vi "to string array.vi"(8 "error in (no error)":errorcluster, 11 "module configuration in":refnum<class "Daqmx Module configuration.lvclass">) -> (0 "error out":errorcluster, 1 "Array":string[][](array[string]), 2 "version":string, 3 "module configuration out":refnum<class "Daqmx Module configuration.lvclass">)   [LabVIEW 2014, in "DAQmx Module Configuration.lvclass"]
uses:
  Daqmx Module configuration.lvclass
  Daqmx Module configuration.lvclass/Daqmx Module configuration.ctl
  <vilib>/NI/Tag Bus/tag/tag descriptor.lvclass/tag descriptor.ctl
  <vilib>/NI/Tag Bus Module Framework/module configuration/TBM module configuration.lvclass
  <vilib>/NI/Tag Bus/tag/tag descriptor.lvclass
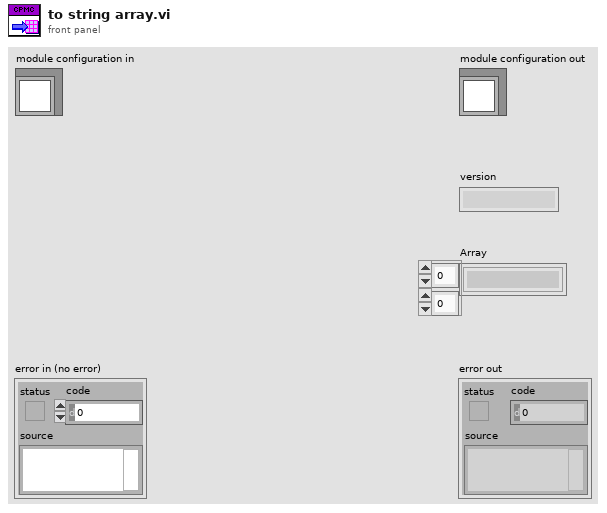
[diagram p1: front panel]
types:
  T1 = typedef "DAQmx Module Configuration.lvclass/Line.ctl" = cluster{"channel":refnum<class "TBM channel.lvclass">, "Physical Channel":string, "Measurement Type":T2, "Parameters":T3}
  T2 = typedef "DAQmx Module Configuration.lvclass/Measurement Type.ctl" = enum16{"Digital Input", "Digital Output", "Voltage Input", "Voltage Output", "Current Input", "Current Output", "RTD", "Thermocouple", "Strain"}
  T3 = typedef "DAQmx Module Configuration.lvclass/Parameters.ctl" = cluster{"Digital Config":cluster{"Invert Lines?":bool}, "Voltage Config":cluster{"Maximum Value (V)":dbl, "Minimum Value (V)":dbl, "in terminal configuration (V)":i32, "out terminal configuration (V)":i32}, "Current Config":cluster{"Maximum Value (A)":dbl, "Minimum Value (A)":dbl, "shunt resistor location":i32, "input terminal configuration (C)":i32, "external shunt resistor value":dbl}, "RTD Config":cluster{"Maximum Value (°C)":dbl, "Minimum Value (°C)":dbl, "resistance configuration":i32, "r0":dbl, "current excitation value":dbl, "rtd type":i32, "current excitation source":i32}, "Thermocouple Config":cluster{"Minimum Value (C)":dbl, "Maximum Value (C)":dbl, "thermocouple type":i32, "cjc source":i32, "cjc value":dbl}, "Strain Config":cluster{"Maximum Value":dbl, "Minimum Value":dbl, "bridge information":cluster{"strain configuration":i32, "lead wire resistance":dbl, "initial bridge voltage":dbl, "voltage excitation source":i32, "voltage excitation value":dbl}, "strain gage information":cluster{"gage factor":dbl, "nominal gage resistance":dbl, "poisson ratio":dbl}}}
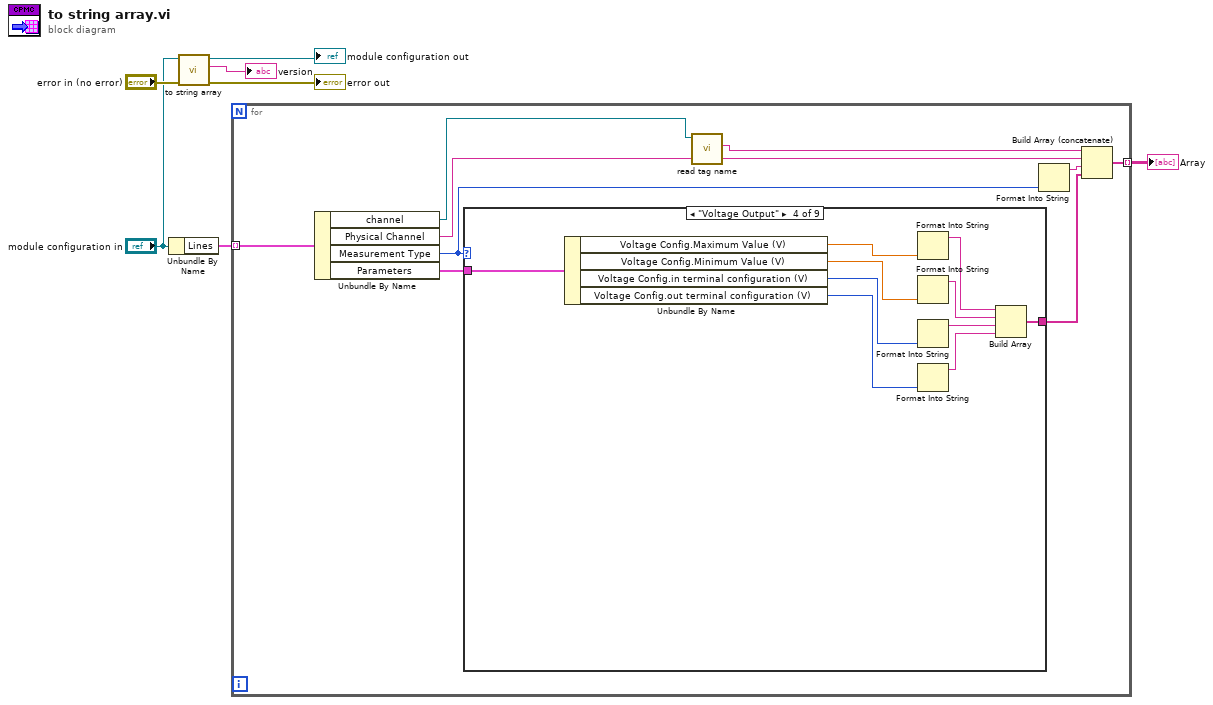
[diagram p0: block diagram]
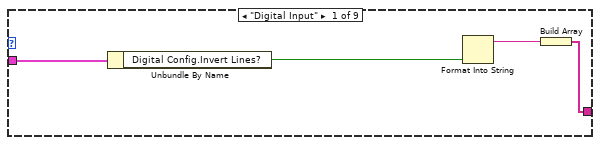
[diagram p2: hidden frame]
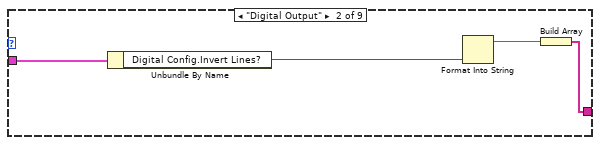
[diagram p3: hidden frame]
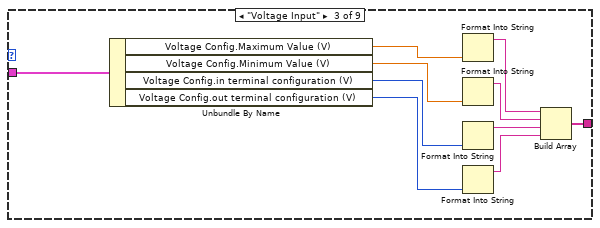
[diagram p4: hidden frame]
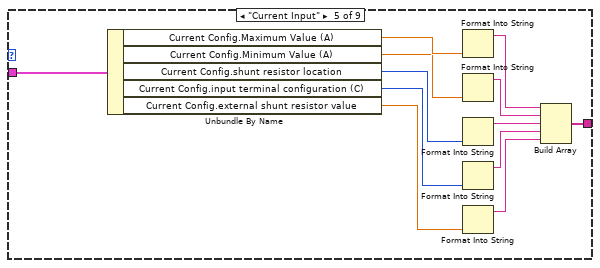
[diagram p5: hidden frame]
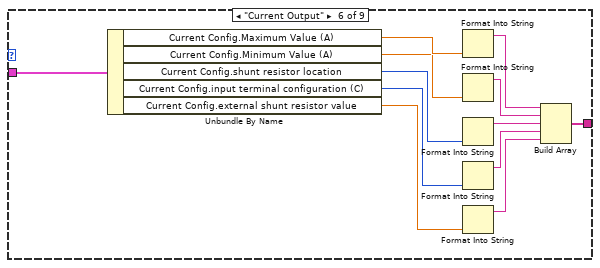
[diagram p6: hidden frame]
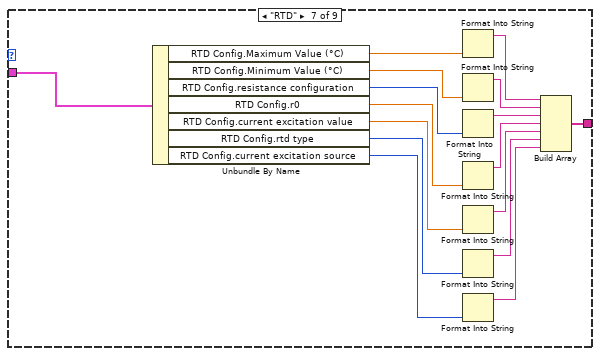
[diagram p7: hidden frame]
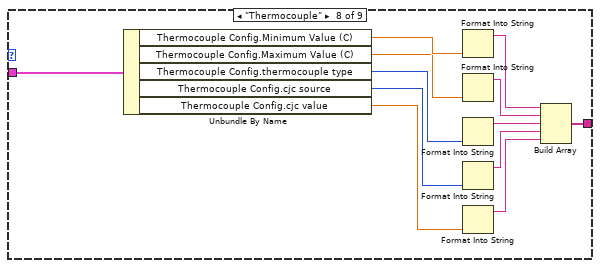
[diagram p8: hidden frame]
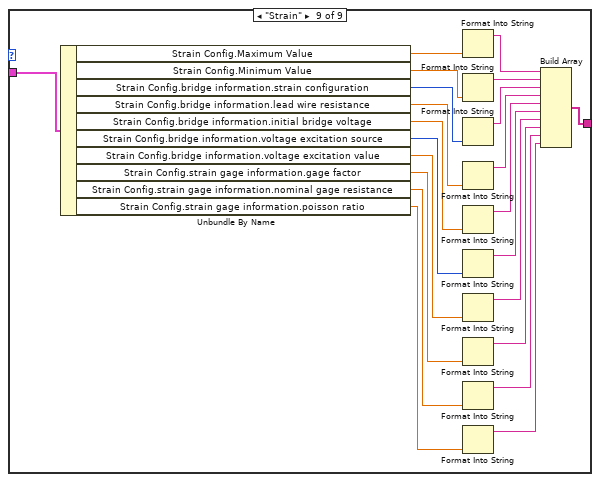
[diagram p9: hidden frame]
diagram:
  n1 = Unbundle By Name("module configuration in") -> ("Lines"=w2:T1[])
  n2 = call-parent "to string array.vi"("error in (no error)"="error in (no error)", "module configuration in"="module configuration in") -> ("error out"=→"error out":errorcluster, "version"=→"version":string, "module configuration out"=→"module configuration out":refnum<class "Daqmx Module configuration.lvclass">)  [unwired: 6 in, 1 out]
  n3 = for {
    tunnel: [w13] -> w1 mode=indexing
    tunnel: w2 -> [w16] mode=indexing
    n4 = Unbundle By Name(w16) -> ("channel"=w9:refnum<class "TBM channel.lvclass">, "Physical Channel"=w15:string, "Measurement Type"=w12:T2, "Parameters"=w11:T3)
    n5 = case shown="\"Voltage Output\"" w12 {
      tunnel: w11 -> [w20 w24 w34 w44 w56 w68 w84 w96 w118]
      tunnel: [w17 w21 w31 w41 w53 w65 w81 w93 w115] -> w10
      frame "Digital Input" {
        n6 = Unbundle By Name(w20) -> ("Digital Config.Invert Lines?"=w19:bool)
        n7 = Format Into String(w19) -> (resulting string=w18:string)  [unwired: 3 in, 1 out]
        n8 = Build Array(w18) -> (w17:string[])
      }
      frame "Digital Output" {
        n9 = Unbundle By Name(w24) -> ("Digital Config.Invert Lines?"=w23:bool)
        n10 = Format Into String(w23) -> (resulting string=w22:string)  [unwired: 3 in, 1 out]
        n11 = Build Array(w22) -> (w21:string[])
      }
      frame "Voltage Input" {
        n12 = Unbundle By Name(w34) -> ("Voltage Config.Maximum Value (V)"=w33:dbl, "Voltage Config.Minimum Value (V)"=w27:dbl, "Voltage Config.in terminal configuration (V)"=w26:i32, "Voltage Config.out terminal configuration (V)"=w25:i32)
        n13 = Format Into String(w33) -> (resulting string=w32:string)  [unwired: 3 in, 1 out]
        n14 = Format Into String(w27) -> (resulting string=w30:string)  [unwired: 3 in, 1 out]
        n15 = Format Into String(w26) -> (resulting string=w29:string)  [unwired: 3 in, 1 out]
        n16 = Format Into String(w25) -> (resulting string=w28:string)  [unwired: 3 in, 1 out]
        n17 = Build Array(w32, w30, w29, w28) -> (w31:string[])
      }
      frame "Voltage Output" {
        n18 = Unbundle By Name(w44) -> ("Voltage Config.Maximum Value (V)"=w43:dbl, "Voltage Config.Minimum Value (V)"=w37:dbl, "Voltage Config.in terminal configuration (V)"=w36:i32, "Voltage Config.out terminal configuration (V)"=w35:i32)
        n19 = Format Into String(w43) -> (resulting string=w42:string)  [unwired: 3 in, 1 out]
        n20 = Format Into String(w37) -> (resulting string=w40:string)  [unwired: 3 in, 1 out]
        n21 = Format Into String(w36) -> (resulting string=w39:string)  [unwired: 3 in, 1 out]
        n22 = Format Into String(w35) -> (resulting string=w38:string)  [unwired: 3 in, 1 out]
        n23 = Build Array(w42, w40, w39, w38) -> (w41:string[])
      }
      frame "Current Input" {
        n24 = Unbundle By Name(w56) -> ("Current Config.Maximum Value (A)"=w55:dbl, "Current Config.Minimum Value (A)"=w49:dbl, "Current Config.shunt resistor location"=w50:i32, "Current Config.input terminal configuration (C)"=w51:i32, "Current Config.external shunt resistor value"=w52:dbl)
        n25 = Format Into String(w55) -> (resulting string=w54:string)  [unwired: 3 in, 1 out]
        n26 = Format Into String(w49) -> (resulting string=w48:string)  [unwired: 3 in, 1 out]
        n27 = Format Into String(w50) -> (resulting string=w47:string)  [unwired: 3 in, 1 out]
        n28 = Format Into String(w51) -> (resulting string=w46:string)  [unwired: 3 in, 1 out]
        n29 = Format Into String(w52) -> (resulting string=w45:string)  [unwired: 3 in, 1 out]
        n30 = Build Array(w54, w48, w47, w46, w45) -> (w53:string[])
      }
      frame "Current Output" {
        n31 = Unbundle By Name(w68) -> ("Current Config.Maximum Value (A)"=w67:dbl, "Current Config.Minimum Value (A)"=w61:dbl, "Current Config.shunt resistor location"=w62:i32, "Current Config.input terminal configuration (C)"=w63:i32, "Current Config.external shunt resistor value"=w64:dbl)
        n32 = Format Into String(w67) -> (resulting string=w66:string)  [unwired: 3 in, 1 out]
        n33 = Format Into String(w61) -> (resulting string=w60:string)  [unwired: 3 in, 1 out]
        n34 = Format Into String(w62) -> (resulting string=w59:string)  [unwired: 3 in, 1 out]
        n35 = Format Into String(w63) -> (resulting string=w58:string)  [unwired: 3 in, 1 out]
        n36 = Format Into String(w64) -> (resulting string=w57:string)  [unwired: 3 in, 1 out]
        n37 = Build Array(w66, w60, w59, w58, w57) -> (w65:string[])
      }
      frame "RTD" {
        n38 = Unbundle By Name(w84) -> ("RTD Config.Maximum Value (°C)"=w83:dbl, "RTD Config.Minimum Value (°C)"=w80:dbl, "RTD Config.resistance configuration"=w71:i32, "RTD Config.r0"=w79:dbl, "RTD Config.current excitation value"=w78:dbl, "RTD Config.rtd type"=w77:i32, "RTD Config.current excitation source"=w76:i32)
        n39 = Format Into String(w83) -> (resulting string=w82:string)  [unwired: 3 in, 1 out]
        n40 = Format Into String(w80) -> (resulting string=w75:string)  [unwired: 3 in, 1 out]
        n41 = Format Into String(w71) -> (resulting string=w70:string)  [unwired: 3 in, 1 out]
        n42 = Format Into String(w79) -> (resulting string=w69:string)  [unwired: 3 in, 1 out]
        n43 = Format Into String(w78) -> (resulting string=w74:string)  [unwired: 3 in, 1 out]
        n44 = Format Into String(w77) -> (resulting string=w73:string)  [unwired: 3 in, 1 out]
        n45 = Format Into String(w76) -> (resulting string=w72:string)  [unwired: 3 in, 1 out]
        n46 = Build Array(w82, w75, w70, w69, w74, w73, w72) -> (w81:string[])
      }
      frame "Thermocouple" {
        n47 = Unbundle By Name(w96) -> ("Thermocouple Config.Minimum Value (C)"=w95:dbl, "Thermocouple Config.Maximum Value (C)"=w92:dbl, "Thermocouple Config.thermocouple type"=w91:i32, "Thermocouple Config.cjc source"=w90:i32, "Thermocouple Config.cjc value"=w89:dbl)
        n48 = Format Into String(w95) -> (resulting string=w94:string)  [unwired: 3 in, 1 out]
        n49 = Format Into String(w92) -> (resulting string=w88:string)  [unwired: 3 in, 1 out]
        n50 = Format Into String(w91) -> (resulting string=w87:string)  [unwired: 3 in, 1 out]
        n51 = Format Into String(w90) -> (resulting string=w86:string)  [unwired: 3 in, 1 out]
        n52 = Format Into String(w89) -> (resulting string=w85:string)  [unwired: 3 in, 1 out]
        n53 = Build Array(w94, w88, w87, w86, w85) -> (w93:string[])
      }
      frame "Strain" {
        n54 = Unbundle By Name(w118) -> ("Strain Config.Maximum Value"=w117:dbl, "Strain Config.Minimum Value"=w114:dbl, "Strain Config.bridge information.strain configuration"=w113:i32, "Strain Config.bridge information.lead wire resistance"=w112:dbl, "Strain Config.bridge information.initial bridge voltage"=w111:dbl, "Strain Config.bridge information.voltage excitation source"=w110:i32, "Strain Config.bridge information.voltage excitation value"=w104:dbl, "Strain Config.strain gage information.gage factor"=w103:dbl, "Strain Config.strain gage information.nominal gage resistance"=w102:dbl, "Strain Config.strain gage information.poisson ratio"=w101:dbl)
        n55 = Format Into String(w117) -> (resulting string=w116:string)  [unwired: 3 in, 1 out]
        n56 = Format Into String(w114) -> (resulting string=w109:string)  [unwired: 3 in, 1 out]
        n57 = Format Into String(w113) -> (resulting string=w108:string)  [unwired: 3 in, 1 out]
        n58 = Format Into String(w112) -> (resulting string=w107:string)  [unwired: 3 in, 1 out]
        n59 = Format Into String(w111) -> (resulting string=w106:string)  [unwired: 3 in, 1 out]
        n60 = Format Into String(w110) -> (resulting string=w105:string)  [unwired: 3 in, 1 out]
        n61 = Format Into String(w104) -> (resulting string=w100:string)  [unwired: 3 in, 1 out]
        n62 = Format Into String(w103) -> (resulting string=w99:string)  [unwired: 3 in, 1 out]
        n63 = Format Into String(w102) -> (resulting string=w98:string)  [unwired: 3 in, 1 out]
        n64 = Format Into String(w101) -> (resulting string=w97:string)  [unwired: 3 in, 1 out]
        n65 = Build Array(w116, w109, w108, w107, w106, w105, w100, w99, w98, w97) -> (w115:string[])
      }
    }
    n66 = call <vilib>:"read tag name.vi"("system tag in"=w9) -> ("name"=w8:string)  [unwired: 8 in, 2 out]
    n67 = Format Into String(w12) -> (resulting string=w14:string)  [unwired: 3 in, 1 out]
    n68 = Build Array (concatenate)(w8, w15, w14, w10) -> (w13:string[])
  }
  "Array" <- w1
